vi "Write Test Parameters.vi"(10 "Test Parameters":T1 {"Max records per file" min=100 max=1000000; "Cycle profile"."Pause After" min=1.0 max=600.0 format="%.1f"; "Cycle profile"."Force Setpoint" min=-556.0 max=556.0 format="%.1f"; "Number of cycles for complete test" min=1}, 11 "Logger in":refnum<class "Logger.lvclass">) -> (3 "Logger out":refnum<class "Logger.lvclass">)   [LabVIEW 2013, in "Logger.lvclass"]
uses:
  Logger.lvclass
  Configuration/Test Parameters.ctl
  Configuration/CycleProfileConfig.ctl
  Logger.lvclass/Logger.ctl
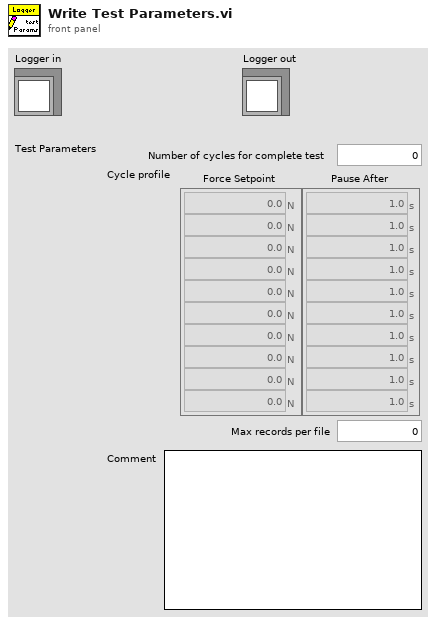
[diagram p1: front panel]
types:
  T1 = typedef "Test Parameters.ctl" = cluster{"Number of cycles for complete test":u32, "Cycle profile":T2, "Max records per file":u32, "Comment":string}
  T2 = typedef "CycleProfileConfig.ctl" = cluster{"Force Setpoint":dbl[unit][], "Pause After":dbl[unit][]}
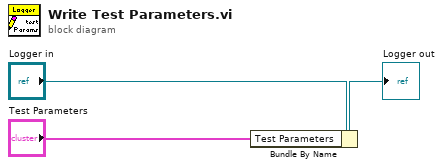
[diagram p0: block diagram]
diagram:
  n1 = Bundle By Name(cluster="Logger in", "Test Parameters"="Test Parameters") -> (→"Logger out":refnum<class "Logger.lvclass">)
